vi "Initialize DCAF INI.vi"(8 "Error In":errorcluster) -> (0 "Error Out":errorcluster)   [LabVIEW 2014, in "Standard Editor.lvlib" / "DCAF INI.lvlib"]
doc: "Opens session to or creates DCAF INI file.\n\n<b>THIS FUNCTION MUST BE CALLED BEFORE ANY INI ACCESSORS</b>"
uses:
  DCAF INI.lvlib
  <vilib>/Utility/config.llb/NI_LVConfig.lvlib
  Standard Editor.lvlib
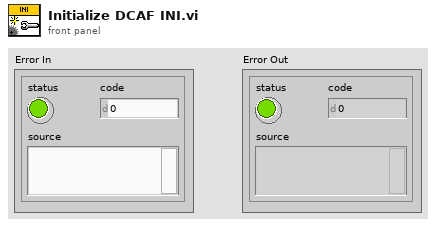
[diagram p1: front panel]
types:
  T1 = typedef "NI_LVConfig.lvlib/Config Data RefNum.ctl" = refnum<k1>
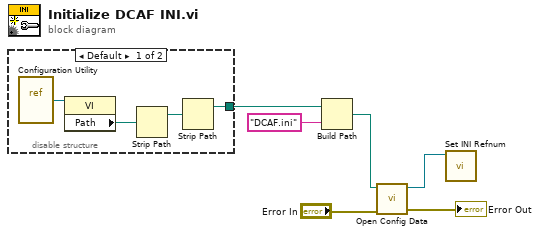
[diagram p0: block diagram]
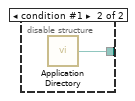
[diagram p2: hidden frame]
diagram:
  n1 = disable-structure shown="Default" {
    disable-tunnel: [w8 w11] -> w3
    frame condition #0 (active) {
      n2 = vi-ref "Configuration Utility.vi"() -> (w10:refnum<vi>)
      n3 = property class="VI"(reference=w10) -> ("Path"=w9:path)  [unwired: 1 in, 2 out]
      n4 = Strip Path(path=w9) -> (stripped path=w7:path)  [unwired: 1 out]
      n5 = Strip Path(path=w7) -> (stripped path=w8:path)  [unwired: 1 out]
    }
    frame condition #1 {
      n6 = call <vilib>:"Application Directory.vi"() -> ("Application Directory"=w11:path)
    }
  }
  n7 = Build Path(base path=w3, name or relative path="DCAF.ini") -> (appended path=w1:path)
  n8 = call <vilib>:"Open Config Data.vi"("error in (no error)"="Error In", "configuration file path"=w1) -> ("error out"=→"Error Out":errorcluster, "refnum"=w4:T1)  [unwired: 7 in, 1 out]
  n9 = call "Set INI Refnum.vi"("INI Refnum In"=w4) -> ()  [unwired: 11 in]
